vi "testGetTel.vi"(8 "error in (no error)":errorcluster) -> (0 "error out":errorcluster)   [LabVIEW 2018]
doc: "Test the getTel.vi"
uses:
  src/TcpServer/TcpServer.lvclass
  src/TcpServer/TcpServer.lvclass/TcpServer.ctl
  src/TcpServerTel/TcpServerTel.lvclass/TcpServerTel.ctl
  <vilib>/addons/_JKI Toolkits/Caraya/classes/Assert/Assert Equal Value_Variant.vi
  src/TcpServerTel/TcpServerTel.lvclass
  <vilib>/addons/_JKI Toolkits/Caraya/classes/Test/Test.lvclass
  <vilib>/addons/_JKI Toolkits/Caraya/classes/Assert/Assert.lvclass
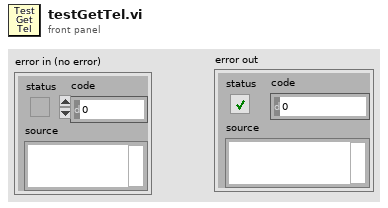
[diagram p1: front panel]
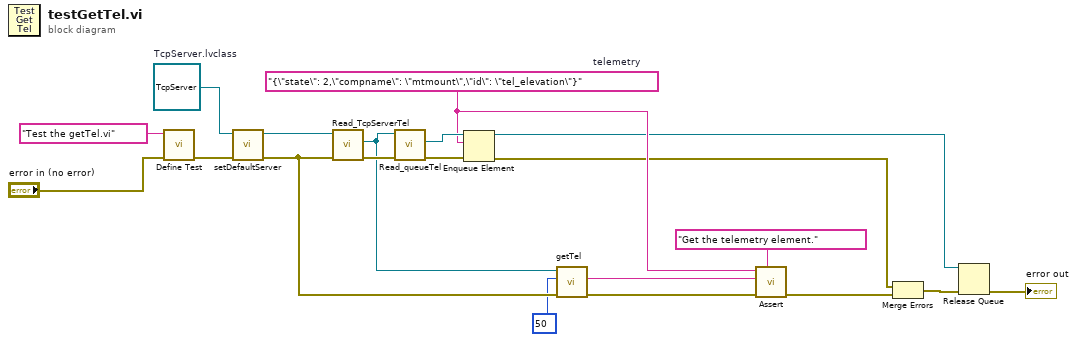
[diagram p0: block diagram]
diagram:
  w9 = "{\"state\": 2,\"compname\": \"mtmount\",\"id\": \"tel_elevation\"}"  # telemetry
  w17 = refnum<class "TcpServer.lvclass"> refnum  # TcpServer.lvclass
  n1 = call <vilib>:"Define Test.vi"("error in (no error)"="error in (no error)", "Label (VI Title)"="Test the getTel.vi") -> ("error out"=w19:errorcluster)  [unwired: 9 in]
  n2 = call "setDefaultServer.vi"("error in (no error)"=w19, "TcpServer.lvclass"=w17) -> ("error out"=w11:errorcluster, "tcpServer out"=w1:refnum<class "TcpServer.lvclass">)  [unwired: 8 in]
  n3 = call "Read_TcpServerTel.vi"("error in (no error)"=w11, "TcpServer in"=w1) -> ("error out"=w14:errorcluster, "TcpServerTel.lvclass"=w2:refnum<class "TcpServerTel.lvclass">)  [unwired: 7 in, 1 out]
  n4 = call "Read_queueTel.vi"("error in (no error)"=w14, "TcpServerTel in"=w2) -> ("error out"=w13:errorcluster, "queueTel"=w12:refnum<queue>)  [unwired: 7 in, 1 out]
  n5 = Enqueue Element(queue=w12, element=w9, error in (no error)=w13) -> (queue out=w5:refnum<queue>, error out=w3:errorcluster)  [unwired: 1 in, 1 out]
  n6 = call "getTel.vi"("error in (no error)"=w11, "telQueueServerTimeout"=50, "tcpServerTel in"=w2) -> ("error out"=w7:errorcluster, "tcpPacket"=w8:string)  [unwired: 5 in, 2 out]
  n7 = call-poly <vilib>:"Assert.vi"("Label"="Get the telemetry element.", "error in (no error)"=w7, "Y"=w8, "X"=w9) -> ("error out"=w15:errorcluster)  [unwired: 7 in]
  n8 = Merge Errors(w3, w15) -> (w4:errorcluster)
  n9 = Release Queue(queue=w5, error in (no error)=w4) -> (error out=→"error out":errorcluster)  [unwired: 1 in, 2 out]
